vi "Write configuration.vi"(8 "error in":errorcluster, 10 "configuration":refnum<class "NISE_CEF_serializable configuration.lvclass">, 11 "TEST EDITOR in":refnum<class "TEST EDITOR.lvclass">) -> (0 "error out":errorcluster, 3 "TEST EDITOR out":refnum<class "TEST EDITOR.lvclass">)   [LabVIEW 2013, in "configuration tests.lvlib" / "TEST EDITOR.lvclass"]
uses:
  TEST EDITOR.lvclass
  <vilib>/NI/Configuration Framework/serializable configuration/NISE_CEF_serializable configuration.lvclass
  module/configuration/TEST CONFIGURATION.lvclass
  TEST EDITOR.lvclass/TEST EDITOR.ctl
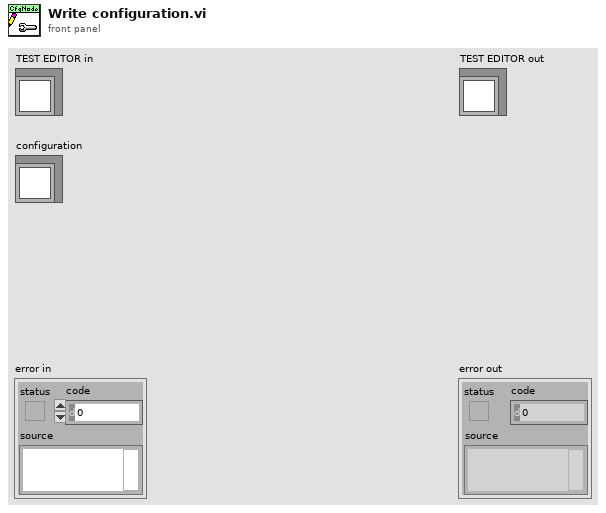
[diagram p1: front panel]
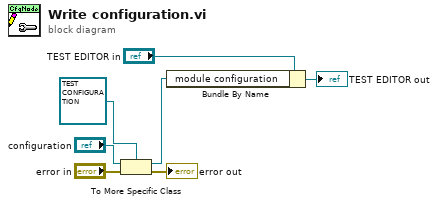
[diagram p0: block diagram]
diagram:
  n1 = To More Specific Class(target class=refnum<class "TEST CONFIGURATION.lvclass"> refnum ("module configuration"), reference="configuration", error in="error in") -> (specific class reference=w4:refnum<class "TEST CONFIGURATION.lvclass">, error out=→"error out":errorcluster)
  n2 = Bundle By Name(cluster="TEST EDITOR in", "module configuration"=w4) -> (→"TEST EDITOR out":refnum<class "TEST EDITOR.lvclass">)
